vi "SCD - Build Recipe Paths.vi"(9 "Selected path":path, 11 "Selected Cookbook":path) -> (0 "error out":errorcluster, 2 "Cookbook Recipes":path[](array[path]), 3 "Valid Check":bool[](array[boolean]), 5 "Cookbook Comments":string="*This is a test comment\r\n*test comment 2\r\n* test comment 3")   [LabVIEW 2014]
doc: "Use this template to build a VI to use as a subVI."
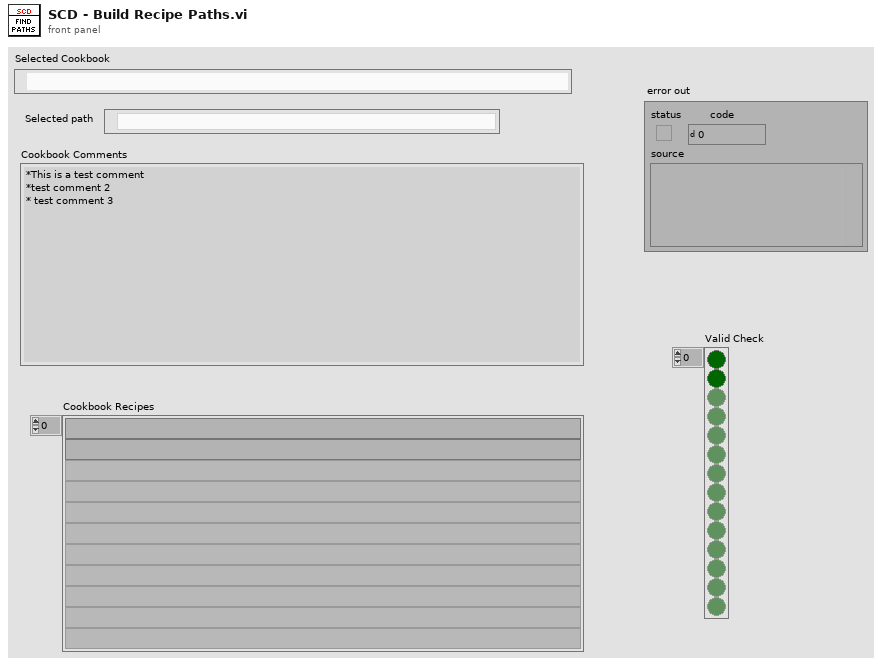
[diagram p1: front panel]
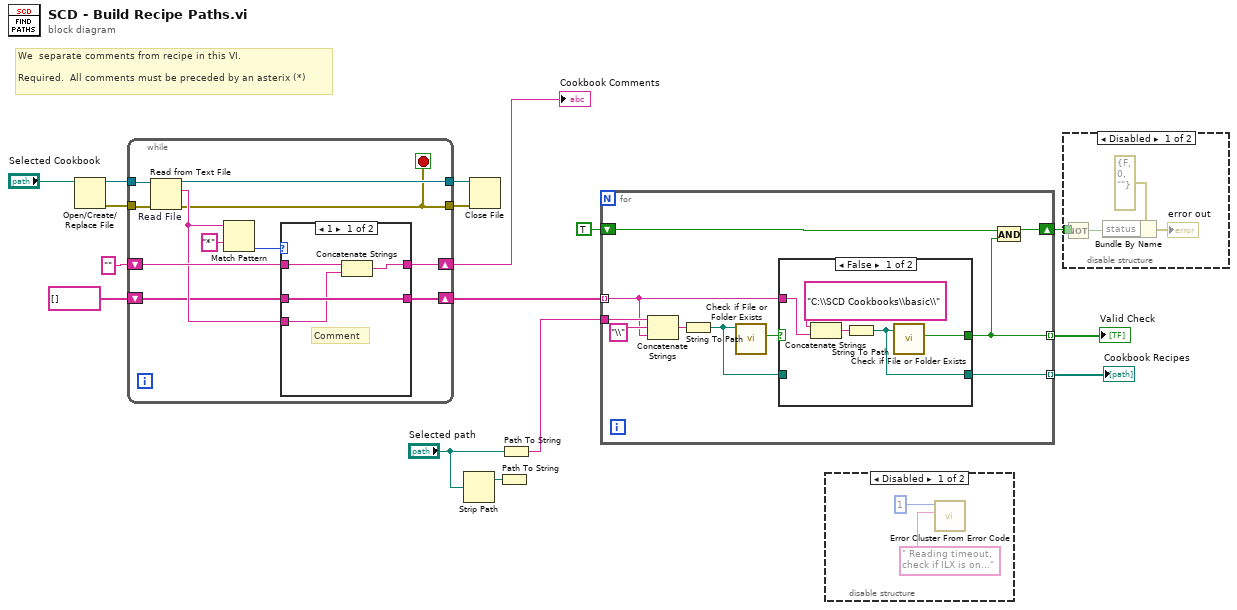
[diagram p0: block diagram]
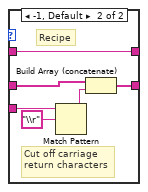
[diagram p5: hidden frame]
diagram:
  # "We  separate comments from recipe in this VI.\n\nRequired.  All comments must be preceded by an asterix (*)"
  n1 = Open/Create/Replace File(file path (use dialog)="Selected Cookbook") -> (refnum out=w16:refnum<file>, error out=w15:errorcluster)  [unwired: 5 in, 1 out]
  n2 = while {
    tunnel: w16 -> [w27]
    tunnel: w15 -> [w26]
    shift-right: [w22] -> w13
    shift-left: "" ("regular expression") -> [w23]
    shift-right: [w19] -> w8
    shift-left: string[] [] ("array of recipes") -> [w20]
    tunnel: [w18] -> w10
    tunnel: [w17] -> w9
    stop <- w17 stop-if-true
    n3 = Read from Text File "Read File"(file (use dialog)=w27, error in=w26) -> (refnum out=w18:refnum<file>, text=w21:string, error out=w17:errorcluster)  [unwired: 3 out]
    n4 = Match Pattern(string=w21, regular expression="*") -> (offset past match=w24:i32)  [unwired: 1 in, 3 out]
    n5 = case shown="1" w24 {
      tunnel: w23 -> [w28 w37]
      tunnel: [w31 w37] -> w22
      tunnel: w21 -> [w29 w34]
      tunnel: w20 -> [w30 w36]
      tunnel: [w30 w35] -> w19
      frame 1 {
        # "Comment"
        n6 = Concatenate Strings(w28, w29) -> (w31:string)
      }
      frame -1, Default {
        # "Cut off carriage \nreturn characters"
        # "Recipe"
        n7 = Match Pattern(string=w34, regular expression="\\r") -> (before substring=w32:string)  [unwired: 1 in, 3 out]
        n8 = Build Array (concatenate)(w36, w32) -> (w35:string[])
      }
    }
  }
  "Cookbook Comments" <- w13
  n9 = Strip Path(path="Selected path") -> (stripped path=w1:path)  [unwired: 1 out]
  n10 = Close File(refnum=w10, error in=w9) -> ()  [unwired: 2 out]
  n11 = Path To String(path=w1) -> ()  [unwired: 1 out]
  n12 = Path To String(path="Selected path") -> (string=w7:string)
  n13 = for {
    tunnel: w8 -> [w41] mode=indexing
    tunnel: w7 -> [w46]
    tunnel: [w38] -> w6 mode=indexing
    tunnel: [w42] -> w5 mode=indexing
    shift-right: [w40] -> w3
    shift-left: TRUE -> [w39]
    n14 = Concatenate Strings(w46, "\\" ("string"), w41) -> (w45:string)
    n15 = String To Path(string=w45) -> (path=w43:path)
    n16 = call <vilib>:"Check if File or Folder Exists.vi"("path"=w43) -> ("file or folder exists?"=w44:bool)  [unwired: 8 in, 2 out]
    n17 = case shown="False" w44 {
      selector: w44 -> [_ w54]
      tunnel: [w49 w54] -> w38
      tunnel: w43 -> [_ w53]
      tunnel: [w48 w53] -> w42
      tunnel: w41 -> [w50 _]
      frame False {
        n18 = Concatenate Strings("C:\\SCD Cookbooks\\basic\\" ("string"), w50) -> (w52:string)
        n19 = String To Path(string=w52) -> (path=w48:path)
        n20 = call <vilib>:"Check if File or Folder Exists.vi"("path"=w48) -> ("file or folder exists?"=w49:bool)  [unwired: 8 in, 2 out]
      }
      frame True {
      }
    }
    n21 = And(x=w39, y=w38) -> (x .and. y?=w40:bool)
  }
  "Cookbook Recipes" <- w5
  "Valid Check" <- w6
  n22 = disable-structure shown="Disabled" {
    frame Disabled {
      n23 = call <vilib>:"Error Cluster From Error Code.vi"("error message (\"\")"=" Reading timeout, check if ILX is on..." ("error message (\"\")"), "error code (0)"=1) -> ()  [unwired: 7 in, 1 out]
    }
    frame Enabled {
    }
  }
  n24 = disable-structure shown="Disabled" {
    disable-tunnel: w3 -> [w58 _]
    frame Disabled {
      n25 = Not(x=w58) -> (.not. x?=w57:bool)
      n26 = Bundle By Name(cluster=errorcluster {"status"=FALSE, "code"=0, "source"=""} ("error out"), "status"=w57) -> (→"error out":errorcluster)
    }
    frame Enabled {
    }
  }
